vi "Get Config Directory Path.vi"() -> (3 "Config Directory Path":path)   [LabVIEW 2020, in "Paths.lvlib"]
uses:
  Paths.lvlib
  <vilib>/Utility/sysdir.llb/System Directory Type.ctl
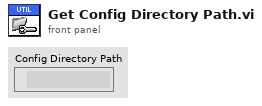
[diagram p1: front panel]
types:
  T1 = typedef "System Directory Type.ctl" = i32
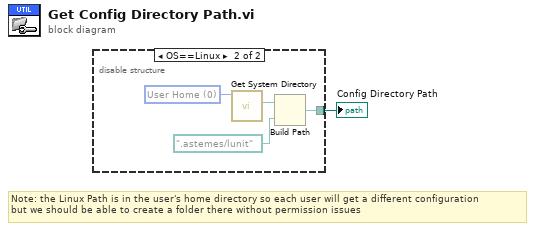
[diagram p0: block diagram]
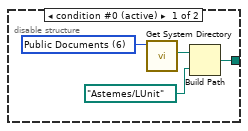
[diagram p2: hidden frame]
diagram:
  # "Note: the Linux Path is in the user's home directory so each user will get a different configuration \nbut we should be able to create a folder there without permission issues"
  n1 = disable-structure shown="OS==Linux" {
    disable-tunnel: [w5 w6] -> w1
    frame condition #0 (active) {
      w4 = T1 6 items=["User Home"=0, "User Desktop"=1, "User Documents"=2, "User Application Data"=3, "User Preferences"=4, "User Temporary"=5, "Public Documents"=6, "Public Application Data"=7, "Public Preferences"=8, "Public Cache"=13, "System Core Libraries"=9, "System Installed Libraries"=10, "Application Files"=11, "Boot Volume Root"=12] ("system directory type")
      n2 = call <vilib>:"Get System Directory.vi"("system directory type"=w4) -> ("system directory"=w2:path)  [unwired: 10 in]
      n3 = Build Path(base path=w2, name or relative path=path "Astemes/LUnit") -> (appended path=w5:path)
    }
    frame condition #1 {
      w9 = T1 0 items=["User Home"=0, "User Desktop"=1, "User Documents"=2, "User Application Data"=3, "User Preferences"=4, "User Temporary"=5, "Public Documents"=6, "Public Application Data"=7, "Public Preferences"=8, "Public Cache"=13, "System Core Libraries"=9, "System Installed Libraries"=10, "Application Files"=11, "Boot Volume Root"=12] ("system directory type")
      n4 = call <vilib>:"Get System Directory.vi"("system directory type"=w9) -> ("system directory"=w7:path)  [unwired: 10 in]
      n5 = Build Path(base path=w7, name or relative path=path ".astemes/lunit") -> (appended path=w6:path)
    }
  }
  "Config Directory Path" <- w1
